vi "rvc 2D Euler to Homogeneous.vi"   [LabVIEW 2013]
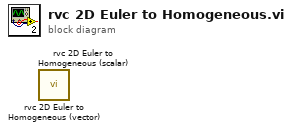
[diagram p0: block diagram]
diagram:
  n1 = call "rvc 2D Euler to Homogeneous (vector).vi"() -> ()  [unwired: 10 in, 2 out]
  n2 = call "rvc 2D Euler to Homogeneous (scalar).vi"() -> ()  [unwired: 10 in, 2 out]
